vi "Connect Control to Connector Pane Terminal.vi"(0 "Connector Pane":refnum<vi>, 1 "Control Ref":refnum<vi>, 2 "Terminal Index":u32, 3 "error in (no error)":errorcluster, 4 "Rule":T1(ring)=enum."Recommended") -> (5 "Connector Pane Out":refnum<vi>, 6 "error out":errorcluster)   [LabVIEW 2018, in "Scripting Tools.lvlib"]
doc: "Connects a control to the connector pane of a VI"
uses:
  Scripting Tools.lvlib
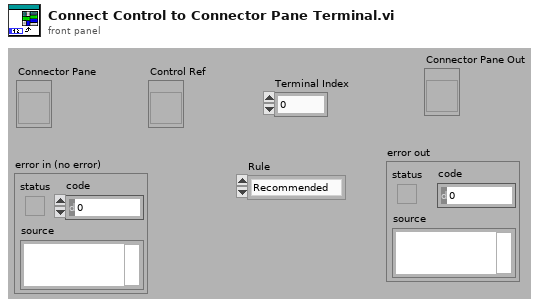
[diagram p1: front panel]
types:
  T1 = enum16{"Invalid Wire Rule", "Required", "Recommended", "Optional", "Dynamic Dispatch"}
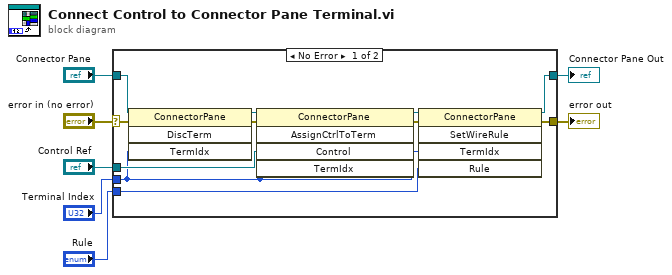
[diagram p0: block diagram]
diagram:
  n1 = case shown="No Error" "error in (no error)" {
    selector: "error in (no error)" -> [w8 w19]
    tunnel: "Connector Pane" -> [w16 w20]
    tunnel: "Control Ref" -> [w15 _]
    tunnel: [w13 w20] -> w5
    tunnel: "Terminal Index" -> [w12 _]
    tunnel: "Rule" -> [w11 _]
    tunnel: [w9 w19] -> w2
    frame No Error {
      n2 = invoke on="Invoke Node" class="ConnectorPane" method="DiscTerm"(reference=w16, error in=w8, "TermIdx"=w12) -> (reference out=w18:refnum<vi>, error out=w17:errorcluster)  [unwired: 1 in, 2 out]
      n3 = invoke on="Invoke Node" class="ConnectorPane" method="AssignCtrlToTerm"(reference=w18, error in=w17, "Control"=w15, "TermIdx"=w12) -> (reference out=w14:refnum<vi>, error out=w10:errorcluster)  [unwired: 1 in, 3 out]
      n4 = invoke on="Invoke Node" class="ConnectorPane" method="SetWireRule"(reference=w14, error in=w10, "TermIdx"=w12, "Rule"=w11) -> (reference out=w13:refnum<vi>, error out=w9:errorcluster)  [unwired: 1 in, 3 out]
    }
    frame Error {
    }
  }
  "error out" <- w2
  "Connector Pane Out" <- w5
